vi "test signal.vi"() -> ()   [LabVIEW 2018]
panel:
  out "Signal Out":waveform(dbl)(graph)
  out "size(s)":i32
  out "Array":dbl[](array[numeric])
  out "Sine":dynamicdata(graph)
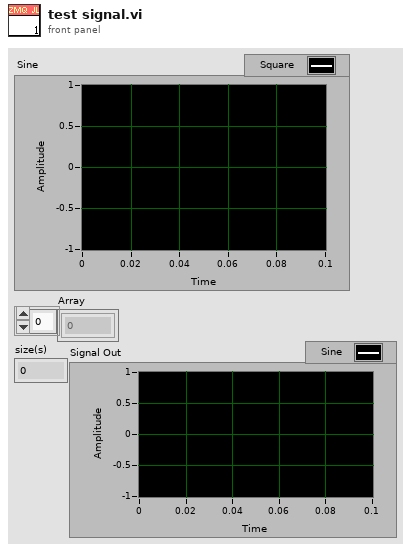
[diagram p1: front panel]
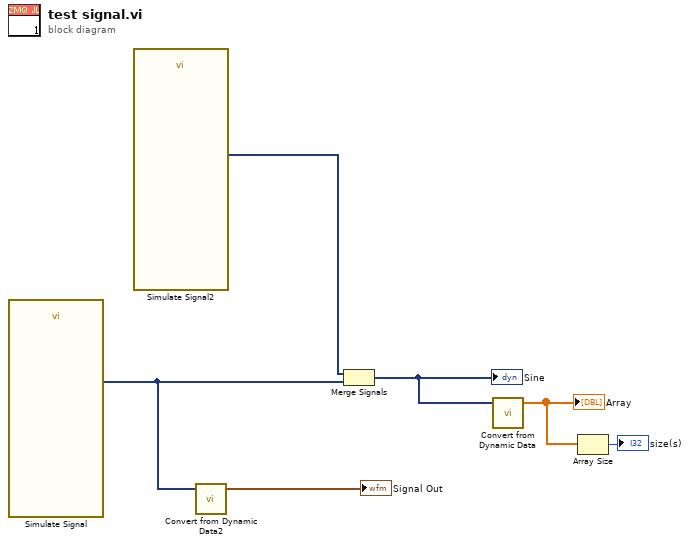
[diagram p0: block diagram]
diagram:
  n1 = call "Simulate Signal"() -> ("Sine"=w2:dynamicdata)  [unwired: 14 in, 1 out]
  n2 = call "Simulate Signal2"() -> ("Square"=w6:dynamicdata)  [unwired: 14 in, 1 out]
  n3 = call "Convert from Dynamic Data2"("Dynamic Data Type"=w2) -> ("Waveform"=→"Signal Out":waveform(dbl))  [unwired: 3 in]
  n4 = Merge Signals(w6, w2) -> (w3:dynamicdata)
  "Sine" <- w3
  n5 = call "Convert from Dynamic Data"("Dynamic Data Type"=w3) -> ("Array"=w5:dbl[])  [unwired: 3 in]
  "Array" <- w5
  n6 = Array Size(array=w5) -> (size(s)=→"size(s)":i32)
